vi "Evaluate Script.vi"(8 "error in (no error)":errorcluster, 10 "Script File Path":path, 11 "Session Handle in":refnum<data-value>) -> (0 "error out":errorcluster, 3 "Session Handle out":refnum<data-value>)   [LabVIEW 2020, in "G-Embedded-Python-Interpreter-Toolkit.lvlib"]
uses:
  G-Embedded-Python-Interpreter-Toolkit.lvlib
  bin/gepit.cp310.32.dll
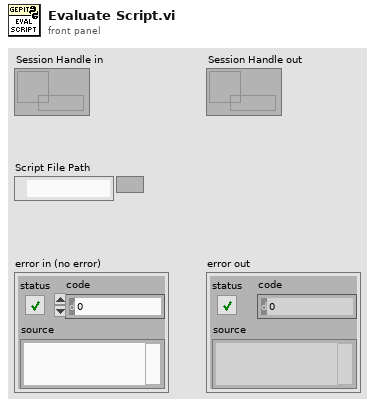
[diagram p1: front panel]
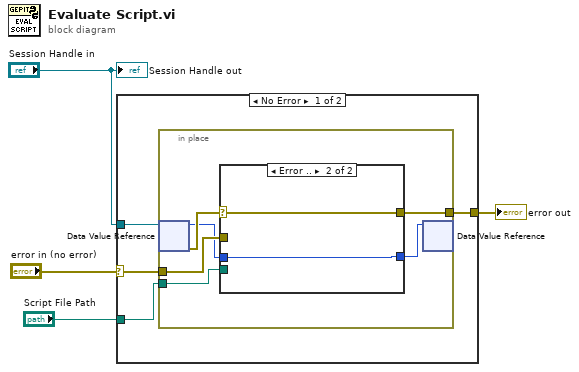
[diagram p0: block diagram]
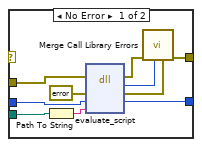
[diagram p2: hidden frame]
diagram:
  n1 = case shown="No Error" "error in (no error)" {
    selector: "error in (no error)" -> [w7 w27]
    tunnel: "Session Handle in" -> [w8 _]
    tunnel: "Script File Path" -> [w6 _]
    tunnel: [w5 w27] -> w1
    frame No Error {
      n2 = in-place {
        in-place-border: w7 -> [w13]
        in-place-border: w6 -> [w10]
        in-place-border: [w9] -> w5
        n3 = in-place-dvr #1(w8) -> (w12:u64, w14:errorcluster)
        n4 = case shown="Error .." w14 {
          selector: w14 -> [_ w25]
          tunnel: w13 -> [w20 _]
          tunnel: w12 -> [w19 w26]
          tunnel: [w18 w26] -> w11
          tunnel: w10 -> [w17 _]
          tunnel: [w15 w25] -> w9
          frame No Error {
            n5 = Path To String(path=w17) -> (string=w16:string)
            n6 = dll-call lib="C:/serenial/libraries/g-embedded-python-interpreter-toolkit/LabVIEW/bin/gepit.cp310.32.dll" fn="evaluate_script"(error in=w20, "Error"=errorcluster {"status"=FALSE, "code"=0, "source"=""} ("error constant"), "Session"=w19, "Script Path"=w16) -> (error out=w23:errorcluster, "return type"=w22:i32, "Error"=w21:errorcluster, "Session"=w18:u64)  [unwired: 3 in, 1 out]
            n7 = call "Merge Call Library Errors.vi"("Call Library Error"=w21, "Return Value"=w22, "error in"=w23) -> ("error out"=w15:errorcluster)  [unwired: 8 in]
          }
          frame Error {
          }
        }
        n8 = in-place-dvr #1(w11) -> ()  [unwired: 2 out]
      }
    }
    frame Error {
    }
  }
  "error out" <- w1
  "Session Handle out" <- "Session Handle in"
